vi "CAD@MotionType__Parameter.vi"(1 "ParamterIn":string) -> (0 "ParamterOut":string)   [LabVIEW 2020]
panel:
  in  "PartName":string(combo)
  in  "Confirm":bool
  # "CAD@MotionType $Parameter"
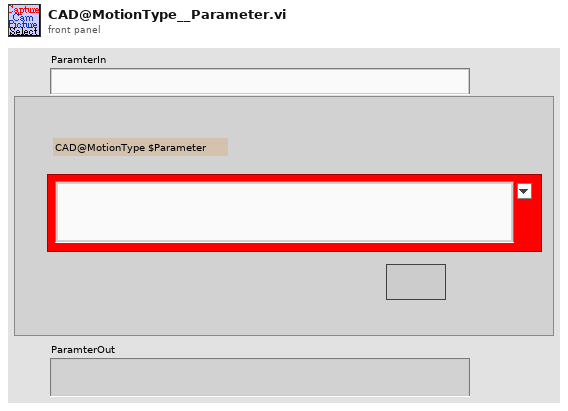
[diagram p1: front panel]
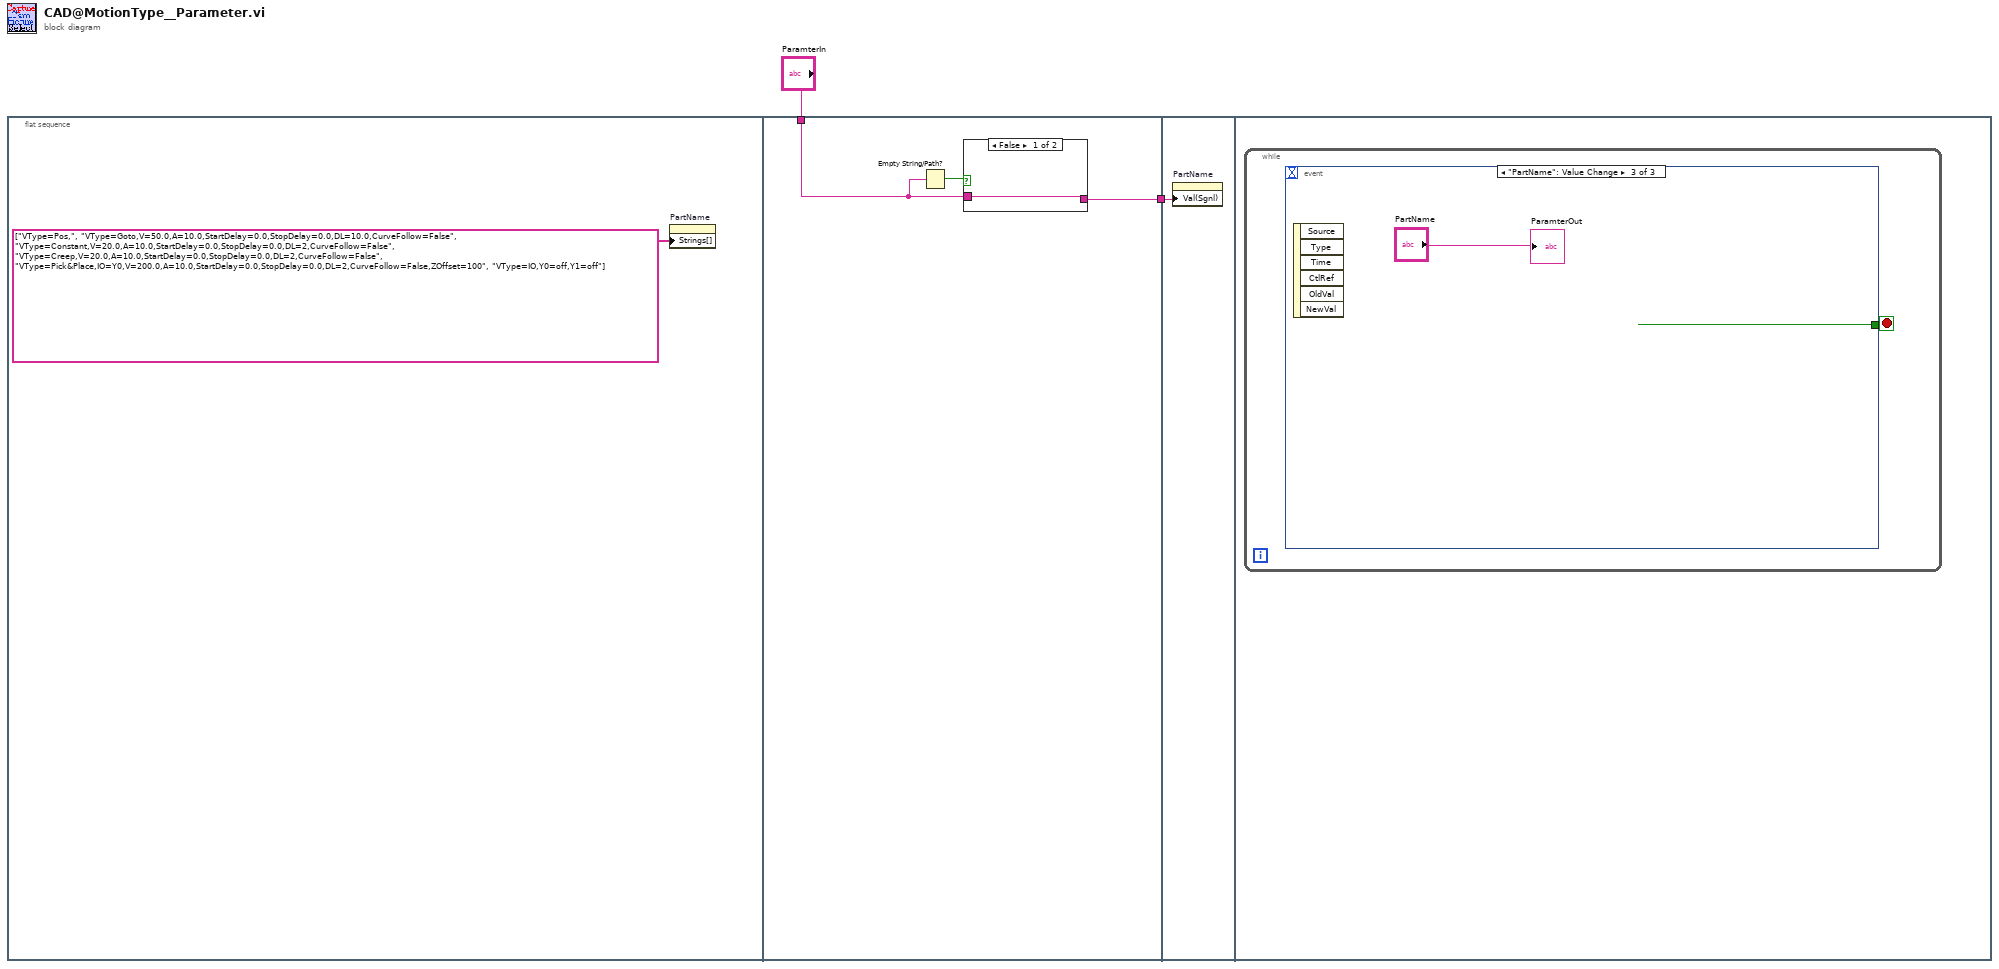
[diagram p0: block diagram]
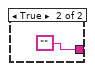
[diagram p2: hidden frame]
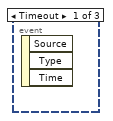
[diagram p3: hidden frame]
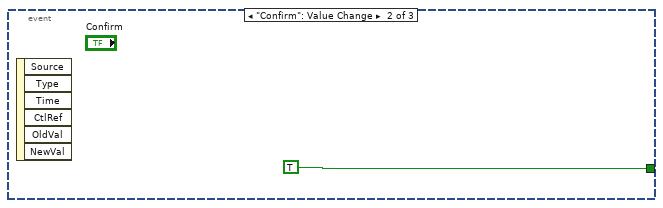
[diagram p4: hidden frame]
diagram:
  n1 = flat-sequence {
    tunnel: "ParamterIn" -> [w4]
    tunnel: [w5] -> w1
    tunnel: w1 -> [w9]
    frame #0 {
      n2 = property on="PartName" class="CmbBox"("Strings[]"=string[] ["VType=Pos,", "VType=Goto,V=50.0,A=10.0,StartDelay=0.0,StopDelay=0.0,DL=10.0,CurveFollow=False", "VType=Constant,V=20.0,A=10.0,StartDelay=0.0,StopDelay=0.0,DL=2,CurveFollow=False", "VType=Creep,V=20.0,A=10.0,StartDelay=0.0,StopDelay=0.0,DL=2,CurveFollow=False", "VType=Pick&Place,IO=Y0,V=200.0,A=10.0,StartDelay=0.0,StopDelay=0.0,DL=2,CurveFollow=False,ZOffset=100", "VType=IO,Y0=off,Y1=off"] ("Strings []")) -> ()  [unwired: 2 in, 2 out]
    }
    frame #1 {
      n3 = Empty String/Path?(string/path=w4) -> (empty?=w6:bool)
      n4 = case shown="False" w6 {
        tunnel: [w7 ""] -> w5
        tunnel: w4 -> [w7 _]
        frame False {
        }
        frame True {
        }
      }
    }
    frame #2 {
      n5 = property on="PartName" class="CmbBox"("Val(Sgnl)"=w9) -> ()  [unwired: 2 in, 2 out]
    }
    frame #3 {
      n6 = while {
        stop <- w10 stop-if-true
        n7 = event shown="[2] \"PartName\": Value Change" {
          selector: _ -> [_ _ _]
          dyn-events: _ -> [_ _ _]
          timeout: _ -> [_ _ _]
          tunnel: [_ TRUE _] -> w10
          event Timeout {
            n8 = event-data() -> ()  [unwired: 1 in, 3 out]
          }
          event "Confirm": Value Change {
            n9 = event-data() -> ()  [unwired: 1 in, 6 out]
          }
          event "PartName": Value Change {
            n10 = event-data() -> ()  [unwired: 1 in, 6 out]
            "ParamterOut" <- "PartName"
          }
        }
      }
    }
  }
